vi "auto_light.vi"() -> ()   [LabVIEW 2017]
uses:
  <vilib>/LabVIEW Interface for Arduino/Type Defs/Arduino Resource.ctl
  <vilib>/LabVIEW Interface for Arduino/Type Defs/Board Type.ctl
  <vilib>/LabVIEW Interface for Arduino/LabVIEW Interface for Arduino.lvlib
panel:
  out "机电控制资源1":T1={"VISA resource"="", "Board Type"=enum."Uno", "Connection Type"=enum."USB / Serial", "Bytes Per Packet (15)"=15} caption="机电控制资源"
  out "机电控制报错1":errorcluster caption="机电控制报错"
  in  "?":enum32{"匀光", "标定", "传感器校准", "参数"}(tab)
  in  "红光":bool
  in  "退出程序":bool
  in  "连接":bool
  in  "SENSOR":refnum<visa-resource-name>
  in  "PWM2":u8=70
  in  "PWM3":u8=70
  in  "PWM1":u8=70
  in  "PWM5":u8=70
  in  "PWM4":u8=70
  in  "PWM6":u8=70
  in  "PWM7":u8=70
  in  "PWM8":u8=70
  in  "PWM9":u8=70
  out "光强2":dbl format="%#.2f"
  out "光强1":dbl format="%#.2f"
  out "光强3":dbl format="%#.2f"
  out "光强4":dbl format="%#.2f"
  out "光强5":dbl format="%#.2f"
  out "光强6":dbl format="%#.2f"
  out "光强7":dbl format="%#.2f"
  out "光强8":dbl format="%#.2f"
  out "光强9":dbl format="%#.2g"
  in  "目标光强":dbl
  in  "紫光":bool
  in  "自动匀光":bool
  out "平均光强":dbl caption="目标光强"
  in  "取消匀光":bool
  in  "精度":dbl caption="目标光强"
  in  "LIGHT":refnum<visa-resource-name>
  in  "开始标定":bool
  out "进度条":string
  out "c":string
  out "b":string
  out "a":string
  out "?":string
  out "?":string
  out "?":string
  out "?":string
  out "?":string
  out "?":string
  out "?":string
  out "?":string
  out "?":string
  out "?":string
  out "?":string
  out "?":string
  out "?":string
  out "?":string
  out "?":string
  out "?":string
  out "?":string
  out "?":string
  out "?":string
  out "?":string
  out "?":string
  out "?":string
  out "?":string
  out "?":string
  out "c":string
  out "b":string
  out "a":string
  out "?":string
  out "?":string
  out "?":string
  out "?":string
  out "?":string
  out "?":string
  out "?":string
  out "?":string
  out "?":string
  out "?":string
  out "?":string
  out "?":string
  out "?":string
  out "?":string
  out "?":string
  out "?":string
  out "?":string
  out "?":string
  out "?":string
  out "?":string
  out "?":string
  out "?":string
  out "?":string
  out "?":string
  out "?":string
  out "?":string
  out "?":string
  out "?":string
  out "?":string
  out "?":string
  out "?":string
  out "?":string
  out "?":string
  out "c":string
  out "b":string
  out "a":string
  out "?":string
  out "?":string
  out "?":string
  out "?":string
  out "?":string
  out "?":string
  out "?":string
  out "?":string
  out "?":string
  out "?":string
  out "?":string
  out "?":string
  out "?":string
  out "?":string
  out "?":string
  out "?":string
  out "?":string
  out "?":string
  out "?":string
  out "?":string
  out "?":string
  out "?":string
  out "?":string
  out "?":string
  out "?":string
  out "?":string
  out "?":string
  out "?":string
  out "?":string
  out "?":string
  out "?":string
  out "?":string
  out "?":string
  out "c":string
  out "b":string
  out "a":string
  out "?":string
  out "?":string
  out "?":string
  out "?":string
  out "?":string
  out "?":string
  out "?":string
  out "?":string
  out "?":string
  in  "红光能量（0-255）":u8=255
  in  "红光PWM Pin":u8=11
  out "PWM Pins 4":u8[](array[numeric])=[8, 9, 10] caption="PWM Pins 3"
  out "PWM Pins 5":u8[](array[numeric])=[5, 6, 7] caption="PWM Pins 2"
  out "PWM Pins 6":u8[](array[numeric])=[2, 3, 4] caption="PWM Pins"
  # "S25"
  # "S13"
  # "S1"
  # "S37"
  # "S26"
  # "S14"
  # "S2"
  # "S27"
  # "S15"
  # "S3"
  # "S28"
  # "S16"
  # "S4"
  # "S29"
  # "S17"
  # "S5"
  # "S30"
  # "S18"
  # "S6"
  # "S31"
  # "S19"
  # "S7"
  # "S32"
  # "S20"
  # "S8"
  # "S33"
  # "S21"
  # "S9"
  # "S34"
  # "S22"
  # "S10"
  # "S35"
  # "S23"
  # "S11"
  # "S36"
  # "S24"
  # "S12"
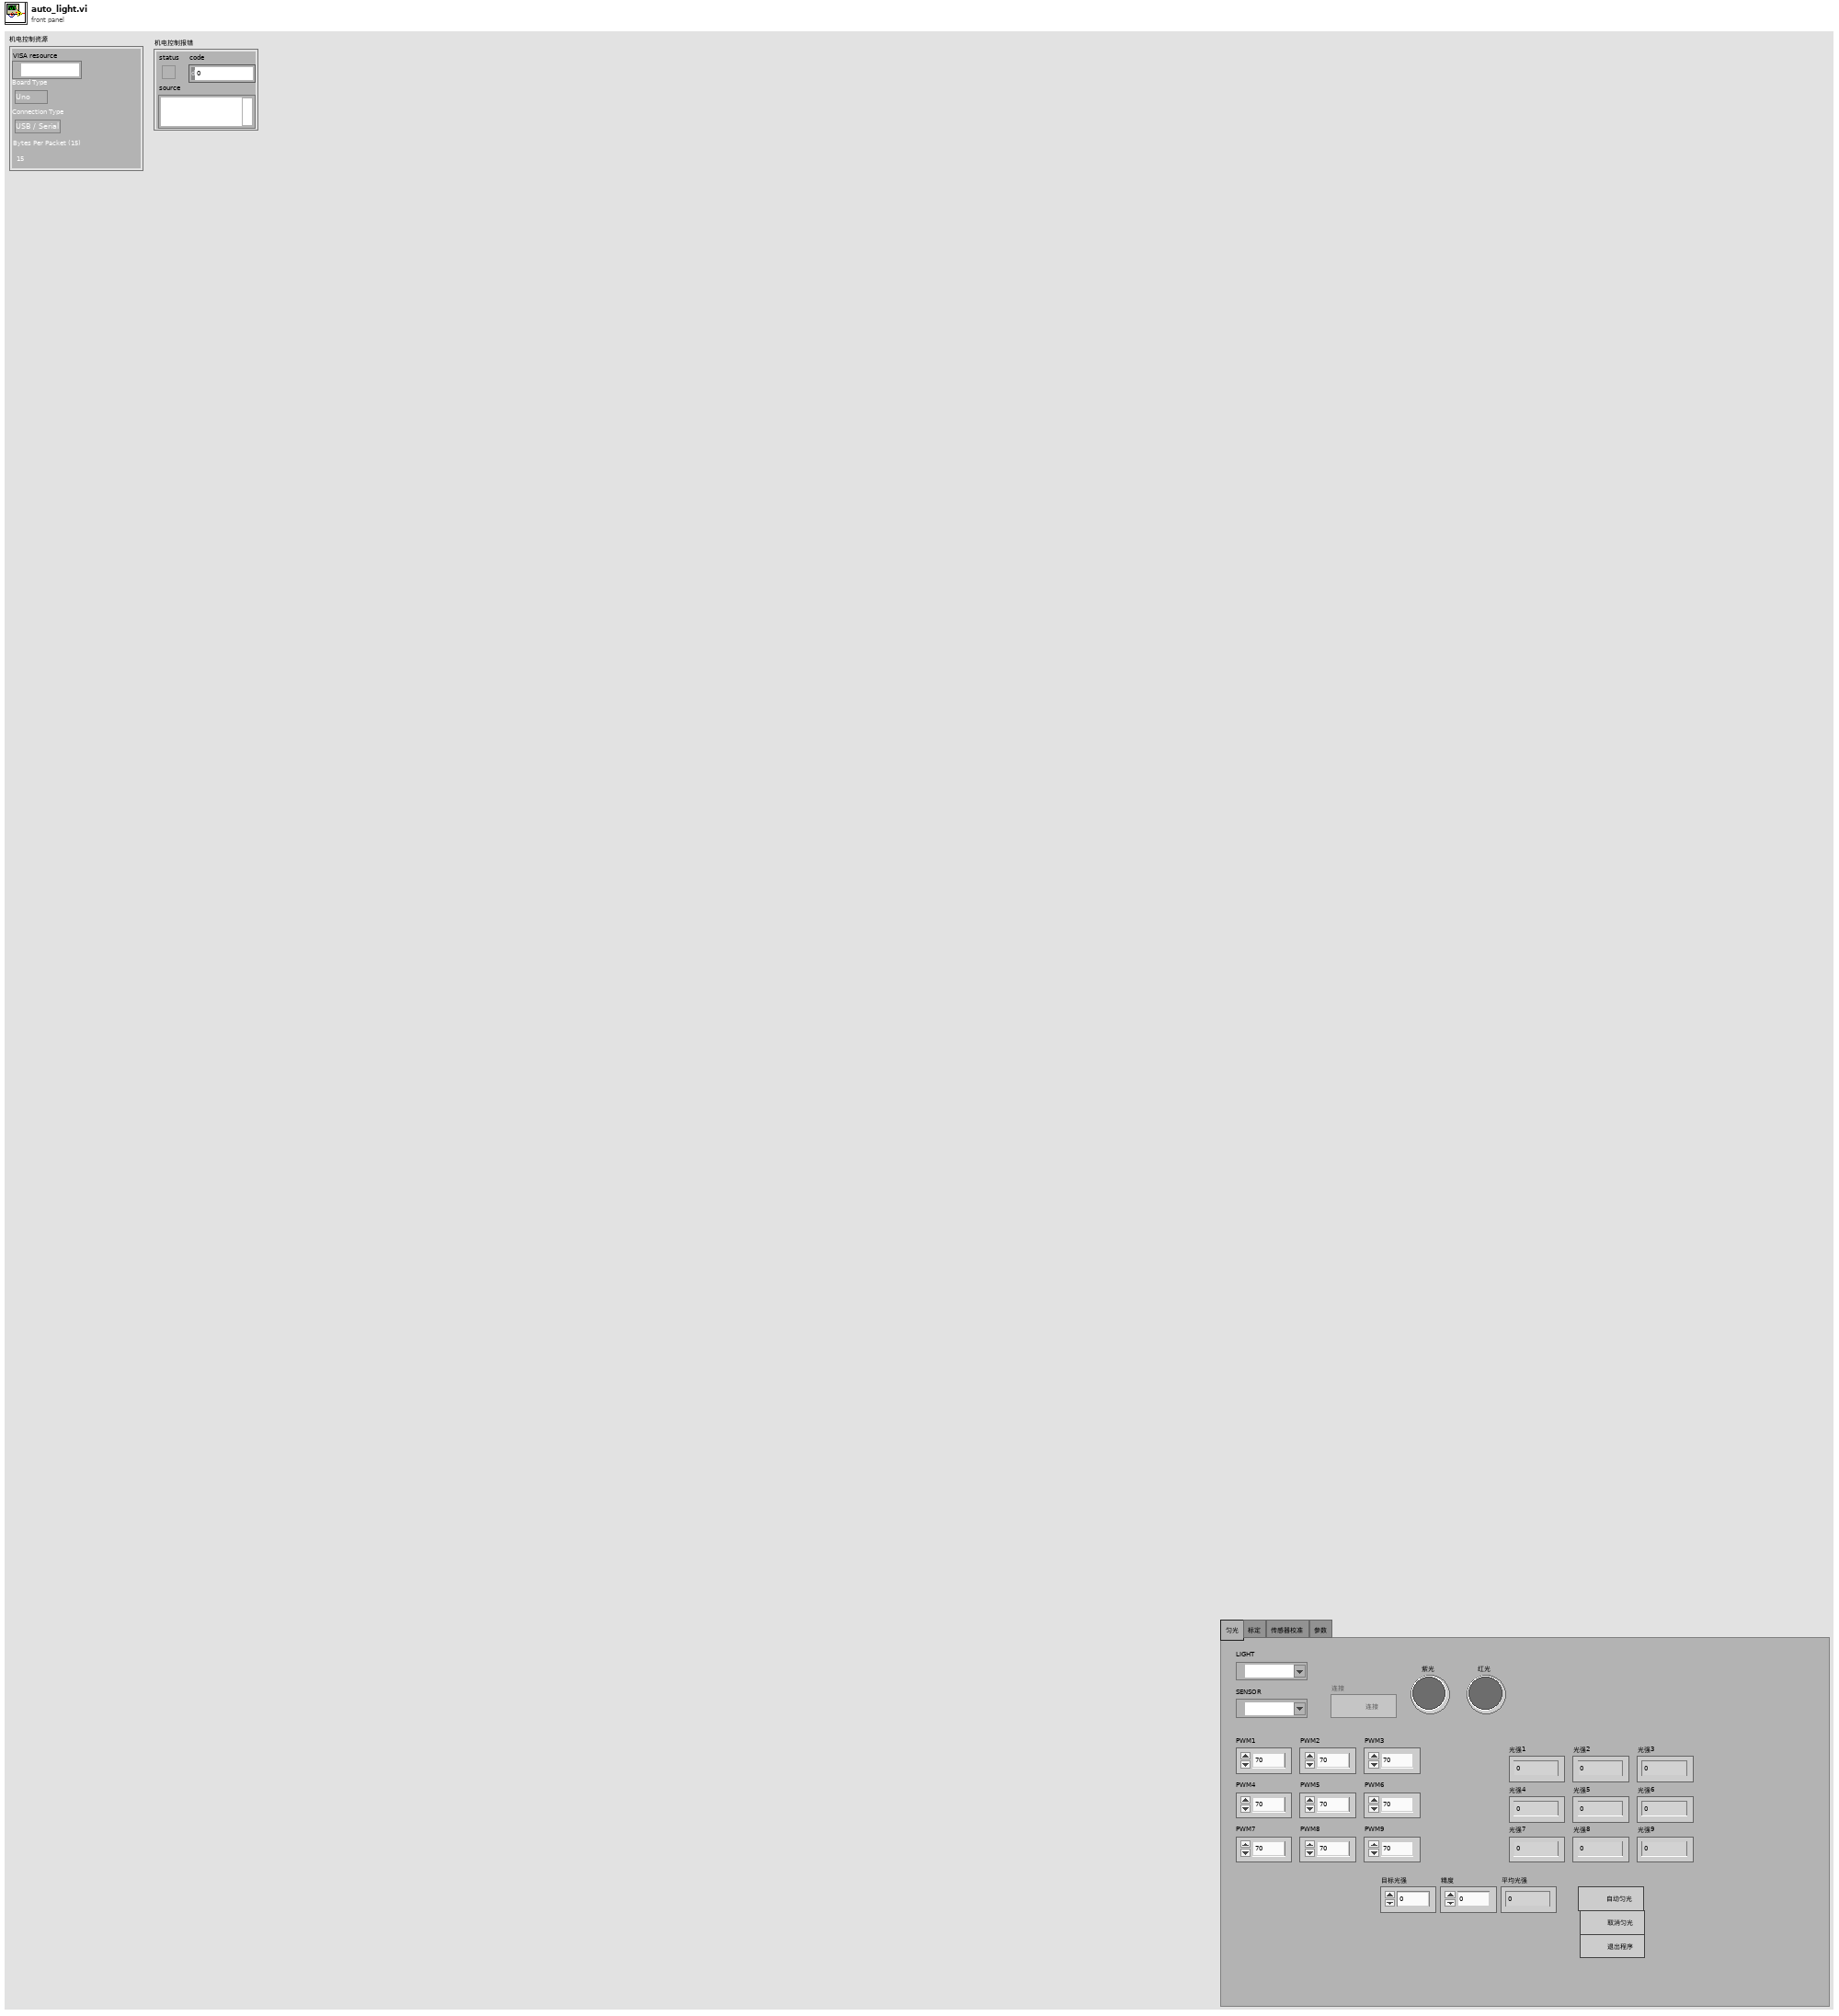
[diagram p1: front panel]
types:
  T1 = typedef "LabVIEW Interface for Arduino.lvlib/Arduino Resource.ctl" = cluster{"VISA resource":refnum<visa-resource-name>, "Board Type":T2, "Connection Type":enum8{"USB / Serial"}, "Bytes Per Packet (15)":u8}
  T2 = typedef "LabVIEW Interface for Arduino.lvlib/Board Type.ctl" = enum16{"Uno", "Dimuelanove w/Atmega 328", "Mega 2560"}
  T3 = enum8{"Enabled", "Disabled", "Disabled and Grayed Out"}
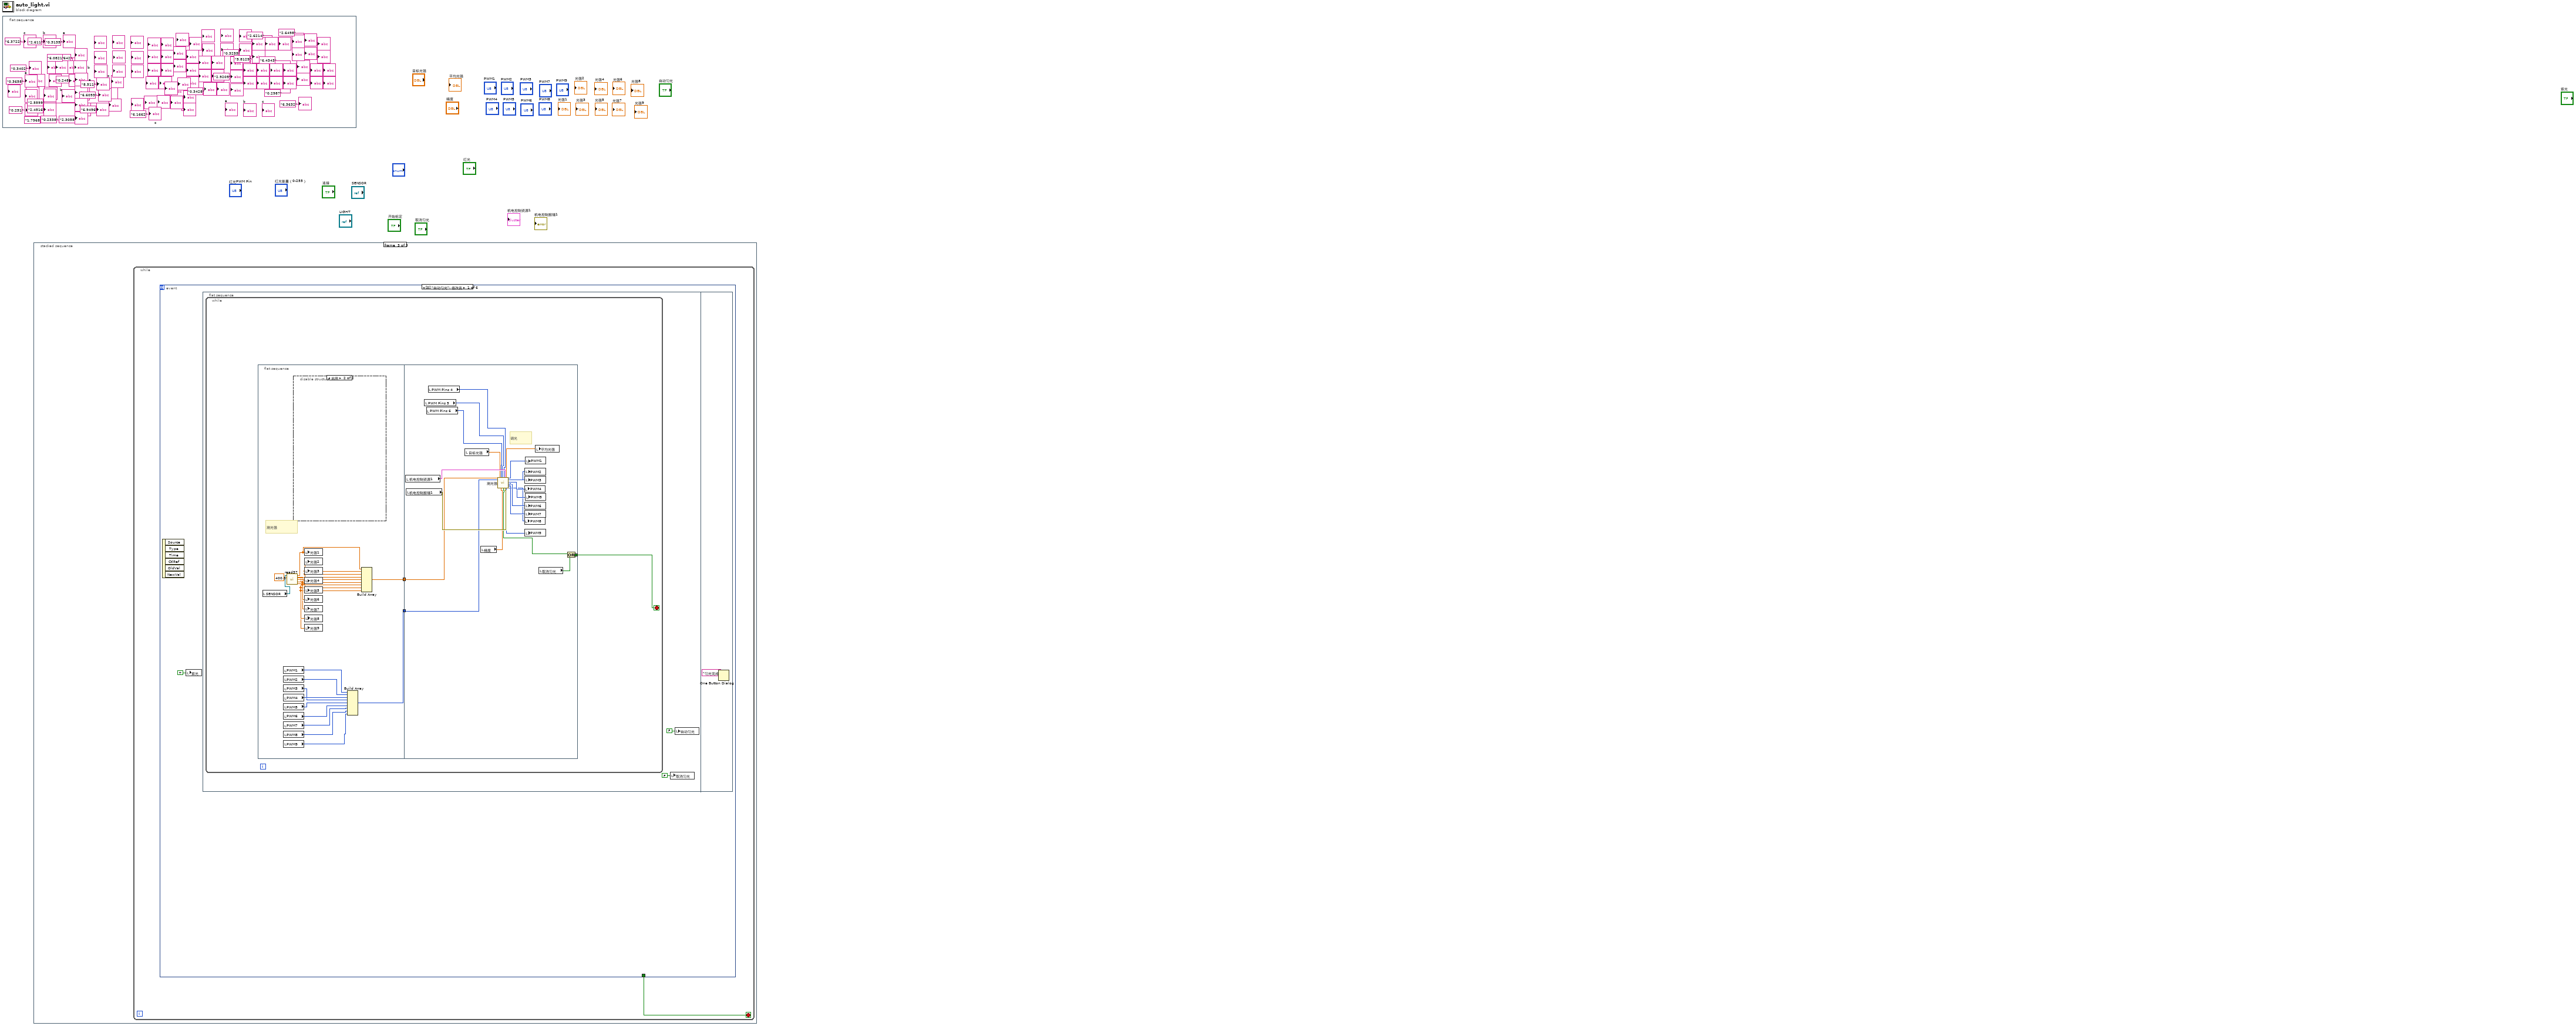
[diagram p0: block diagram]
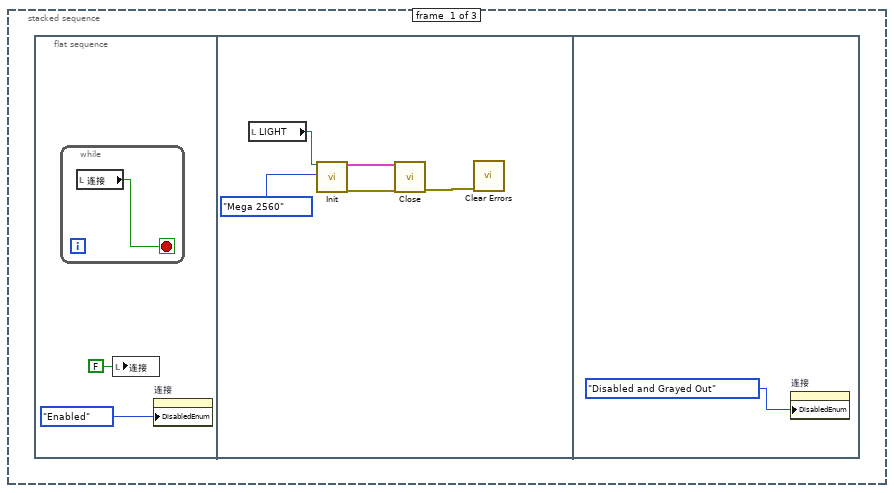
[diagram p2: hidden frame]
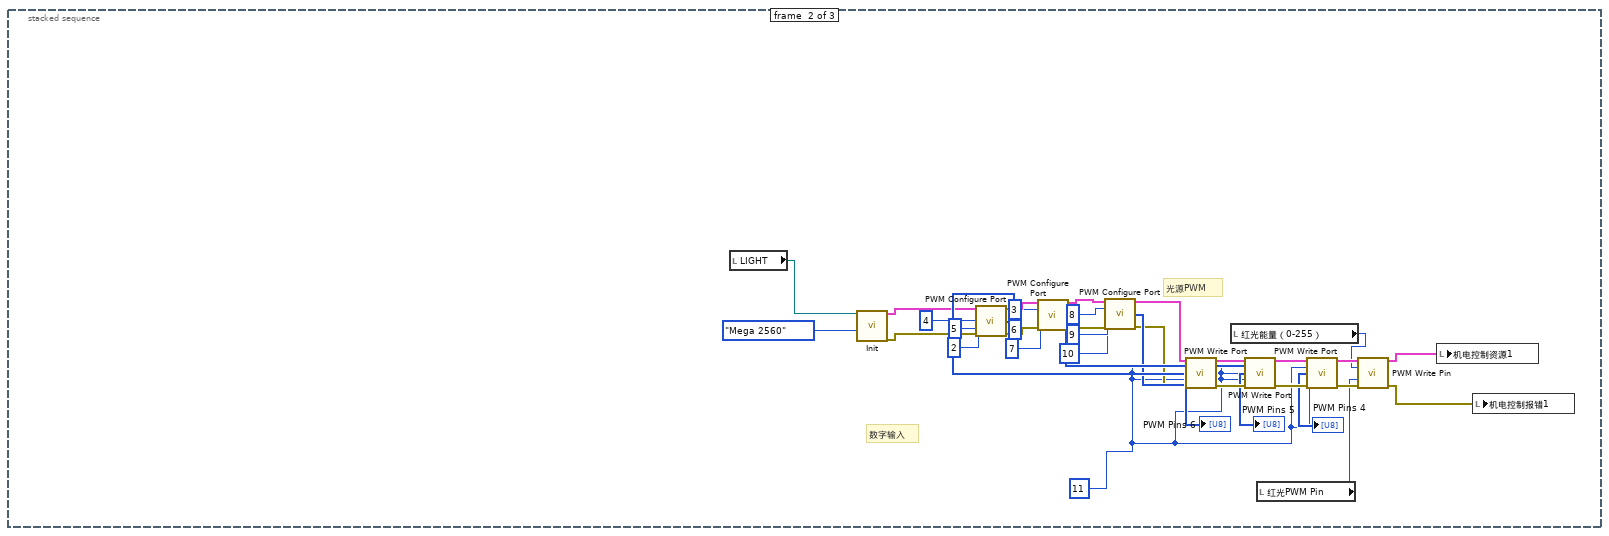
[diagram p3: hidden frame]
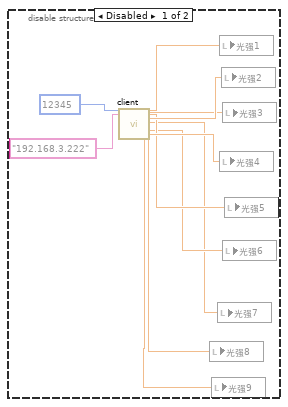
[diagram p4: hidden frame]
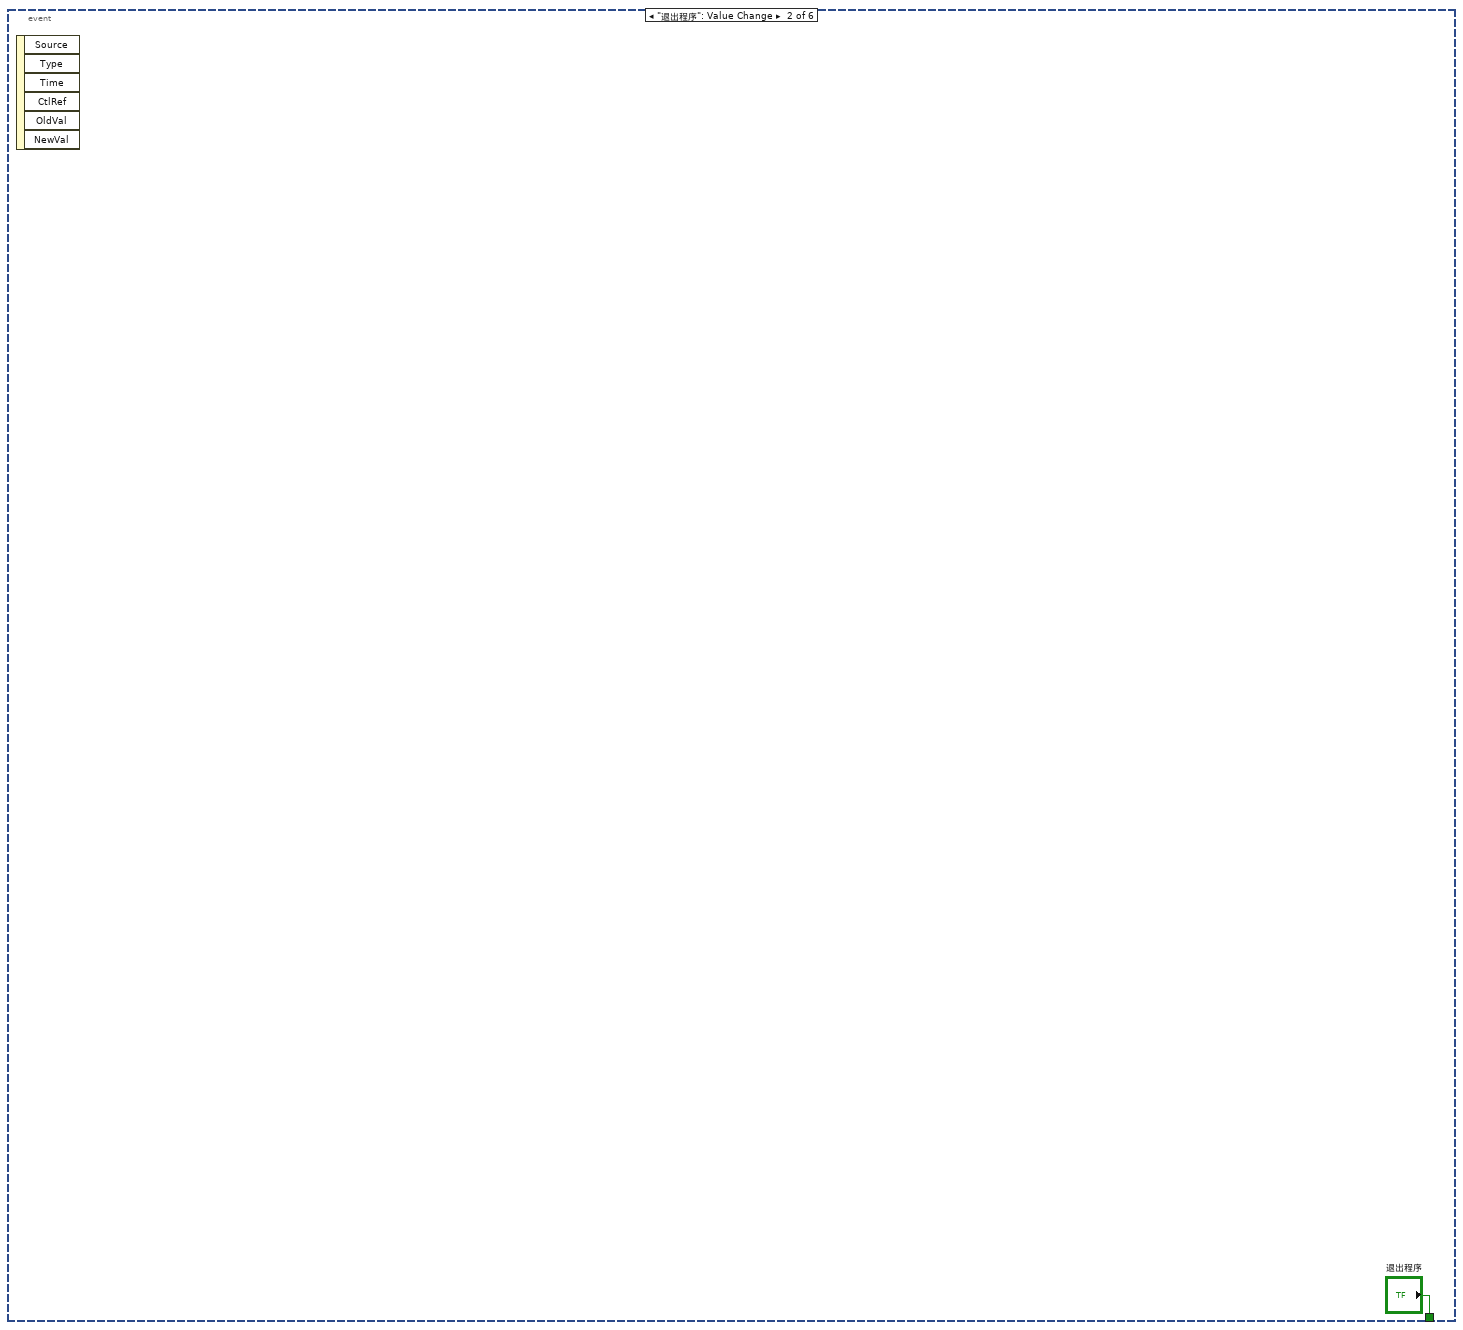
[diagram p5: hidden frame]
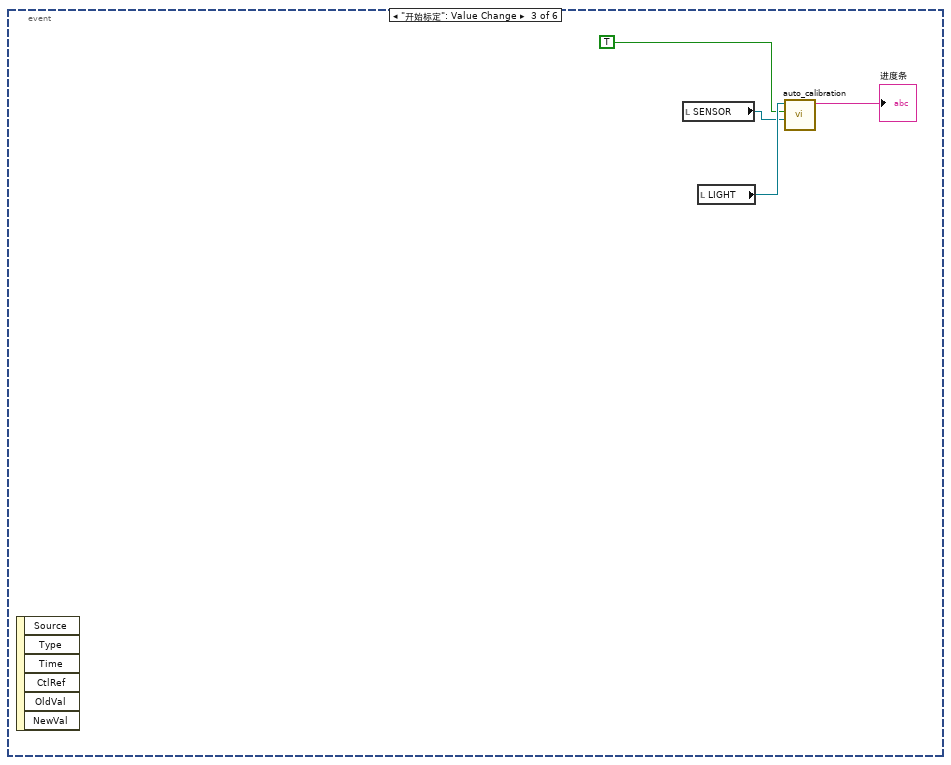
[diagram p6: hidden frame]
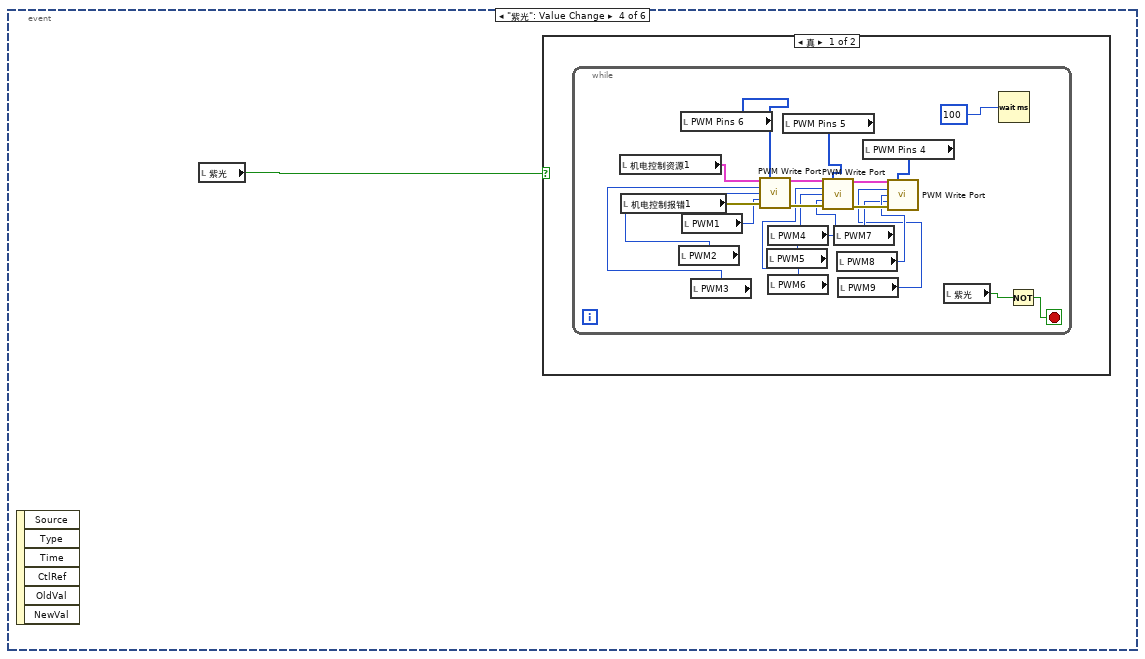
[diagram p7: hidden frame]
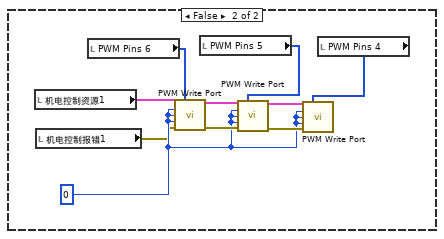
[diagram p8: hidden frame]
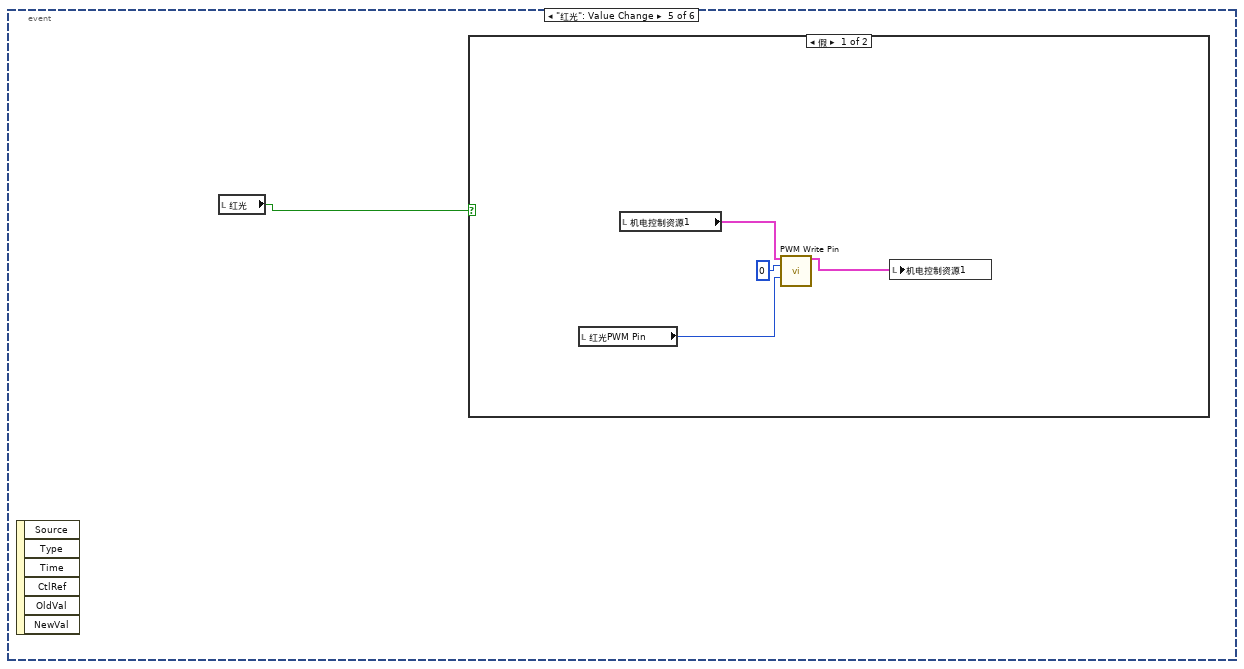
[diagram p9: hidden frame]
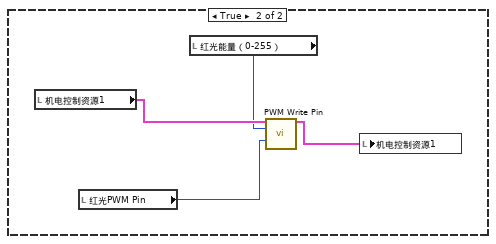
[diagram p10: hidden frame]
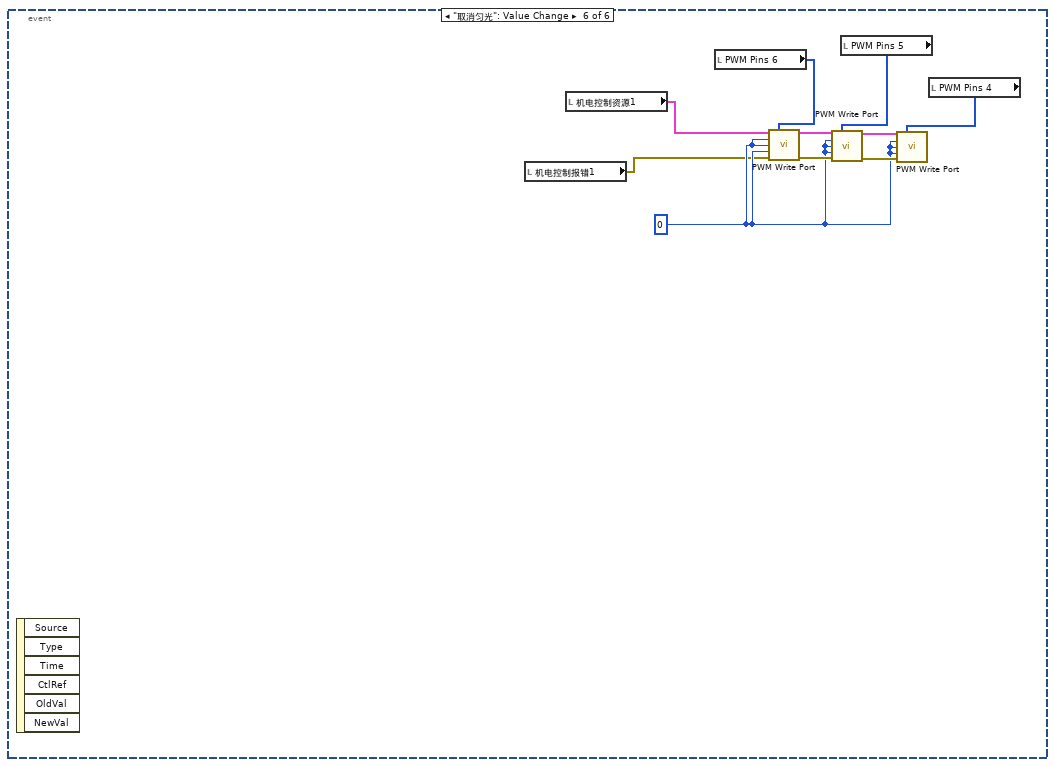
[diagram p11: hidden frame]
diagram:
  n1 = flat-sequence {
    frame #0 {
      "a" <- "0.3135" ("a")
      "c" <- "6.3722" ("c")
      "b" <- "2.611" ("b")
      "a" <- "0.3658" ("a")
      "b" <- "1.7968" ("b")
      "c" <- "8.511" ("c")
      "?" <- "0.251"
      "?" <- "2.4516"
      "?" <- "6.6093"
      "a" <- "0.248" ("a")
      "b" <- "2.7642" ("b")
      "?" <- "2.5599"
      "?" <- "0.3402"
      "?" <- "6.0821"
      "?" <- "0.2338"
      "?" <- "2.3058"
      "?" <- "6.9496"
      "c" <- "6.1662" ("c")
      "?" <- "5.8129"
      "?" <- "2.9209"
      "?" <- "0.3428"
      "?" <- "6.3632"
      "?" <- "2.6214"
      "?" <- "0.3255"
      "?" <- "6.4343"
      "?" <- "2.6498"
      "?" <- "0.2987"
    }
  }
  n2 = stacked-sequence {
    frame #0 {
      n3 = flat-sequence {
        frame #0 {
          n4 = while {
            stop <- w30 stop-if-true
            n5 = local read "连接"() -> (w30:bool)
          }
          n6 = local write "连接"(FALSE ("连接")) -> ()
          n7 = property on="连接" class="Bool (严格)"("DisabledEnum"=T3."Enabled" ("禁用")) -> ()  [unwired: 2 in, 2 out]
        }
        frame #1 {
          n8 = local read "LIGHT"() -> (w31:refnum<visa-resource-name>)
          n9 = call <vilib>:"Init.vi"("VISA resource"=w31, "Board Type (Uno)"=Board_Type."Mega 2560") -> ("Arduino Resource"=w35:T1, "error out"=w34:errorcluster)  [unwired: 16 in]
          n10 = call <vilib>:"Close.vi"("Arduino Resource"=w35, "error in"=w34) -> ("error out"=w33:errorcluster)  [unwired: 13 in]
          n11 = call <vilib>:"Clear Errors.vi"("error in (no error)"=w33) -> ()  [unwired: 5 in, 2 out]
        }
        frame #2 {
          n12 = property on="连接" class="Bool (严格)"("DisabledEnum"=T3."Disabled and Grayed Out" ("禁用")) -> ()  [unwired: 2 in, 2 out]
        }
      }
    }
    frame #1 {
      w40 = 11
      # "数字输入"
      # "光源PWM"
      n13 = local read "LIGHT"() -> (w39:refnum<visa-resource-name>)
      n14 = call <vilib>:"Init.vi"("VISA resource"=w39, "Board Type (Uno)"=Board_Type."Mega 2560") -> ("Arduino Resource"=w42:T1, "error out"=w41:errorcluster)  [unwired: 16 in]
      n15 = call <vilib>:"PWM Configure Port.vi"("Arduino Resource"=w42, "PWM Pin (3)"=u8 4, "PWM Pin (5)"=u8 5, "PWM Pin (6)"=u8 2, "error in"=w41) -> ("Arduino Resource"=w68:T1, "PWM Pins"=w51:u8[], "error out"=w67:errorcluster)  [unwired: 8 in]
      n16 = call <vilib>:"PWM Configure Port.vi"("Arduino Resource"=w68, "PWM Pin (3)"=u8 3, "PWM Pin (5)"=u8 6, "PWM Pin (6)"=u8 7, "error in"=w67) -> ("Arduino Resource"=w53:T1, "PWM Pins"=w50:u8[], "error out"=w52:errorcluster)  [unwired: 8 in]
      n17 = call <vilib>:"PWM Configure Port.vi"("Arduino Resource"=w53, "PWM Pin (3)"=u8 8, "PWM Pin (5)"=u8 9, "PWM Pin (6)"=u8 10, "error in"=w52) -> ("Arduino Resource"=w48:T1, "PWM Pins"=w49:u8[], "error out"=w47:errorcluster)  [unwired: 8 in]
      n18 = call <vilib>:"PWM Write Port.vi"("Arduino Resource"=w48, "PWM Pins"=w51, "PWM 0 (0-255)"=w40, "PWM 1 (0-255)"=w40, "PWM 2 (0-255)"=w40, "error in"=w47) -> ("Arduino Resource"=w60:T1, "PWM Pins"=→"PWM Pins 6":u8[], "error out"=w59:errorcluster)  [unwired: 7 in]
      n19 = local read "红光能量（0-255）"() -> (w43:u8)
      n20 = call <vilib>:"PWM Write Port.vi"("Arduino Resource"=w60, "PWM Pins"=w50, "PWM 0 (0-255)"=w40, "PWM 1 (0-255)"=w40, "PWM 2 (0-255)"=w40, "error in"=w59) -> ("Arduino Resource"=w58:T1, "PWM Pins"=→"PWM Pins 5":u8[], "error out"=w57:errorcluster)  [unwired: 7 in]
      n21 = local read "红光PWM Pin"() -> (w44:u8)
      n22 = call <vilib>:"PWM Write Port.vi"("Arduino Resource"=w58, "PWM Pins"=w49, "PWM 0 (0-255)"=w40, "PWM 1 (0-255)"=w40, "PWM 2 (0-255)"=w40, "error in"=w57) -> ("Arduino Resource"=w46:T1, "PWM Pins"=→"PWM Pins 4":u8[], "error out"=w45:errorcluster)  [unwired: 7 in]
      n23 = call <vilib>:"PWM Write Pin.vi"("Arduino Resource"=w46, "Duty Cycle (0 - 255)"=w43, "PWM Pin (3)"=w44, "error in"=w45) -> ("Arduino Resource"=w38:T1, "error out"=w37:errorcluster)  [unwired: 10 in]
      n24 = local write "机电控制资源1"(w38) -> ()
      n25 = local write "机电控制报错1"(w37) -> ()
    }
    frame #2 {
      n26 = while {
        stop <- w73 stop-if-true
        n27 = event shown="[0] \"自动匀光\": 值改变" {
          selector: _ -> [_ _ _ _ _ _]
          dyn-events: _ -> [_ _ _ _ _ _]
          timeout: _ -> [_ _ _ _ _ _]
          tunnel: [_ "退出程序" _ _ _ _] -> w73
          event "自动匀光": Value Change {
            n28 = event-data() -> ()  [unwired: 1 in, 6 out]
            n29 = local write "紫光"(TRUE ("紫光")) -> ()
            n30 = flat-sequence {
              frame #0 {
                n31 = while {
                  stop <- w79 stop-if-true
                  n32 = flat-sequence {
                    tunnel: [w101] -> w78
                    tunnel: [w100] -> w77
                    tunnel: [w118] -> w79
                    tunnel: w78 -> [w114]
                    tunnel: w77 -> [w113]
                    frame #0 {
                      # "测光强"
                      n33 = local read "SENSOR"() -> (w99:refnum<visa-resource-name>)
                      n34 = local read "PWM1"() -> (w88:u8)
                      n35 = local read "PWM2"() -> (w87:u8)
                      n36 = local read "PWM3"() -> (w86:u8)
                      n37 = local read "PWM4"() -> (w85:u8)
                      n38 = local read "PWM5"() -> (w84:u8)
                      n39 = local read "PWM6"() -> (w83:u8)
                      n40 = local read "PWM7"() -> (w82:u8)
                      n41 = local read "PWM8"() -> (w81:u8)
                      n42 = local read "PWM9"() -> (w80:u8)
                      n43 = call "read37.vi"("VISA资源名称"=w99, "Interval_ms"=400.0) -> ("SENSOR8"=w90:dbl, "SENSOR6"=w92:dbl, "SENSOR1"=w97:dbl, "SENSOR2"=w96:dbl, "SENSOR3"=w95:dbl, "SENSOR4"=w94:dbl, "SENSOR9"=w89:dbl, "SENSOR7"=w91:dbl, "SENSOR5"=w93:dbl)  [unwired: 5 in]
                      n44 = disable-structure shown="启用" {
                        frame Disabled {
                          n45 = call "client.vi"("远程端口或服务名称"=u16 12345, "地址"="192.168.3.222") -> ("num9"=w102:dbl, "num1"=w111:dbl, "num2"=w107:dbl, "num3"=w110:dbl, "num4"=w105:dbl, "num5"=w109:dbl, "num7"=w106:dbl, "num6"=w108:dbl, "num8"=w103:dbl)  [unwired: 17 in]
                          n46 = local write "光强8"(w103) -> ()
                          n47 = local write "光强9"(w102) -> ()
                          n48 = local write "光强7"(w105) -> ()
                          n49 = local write "光强1"(w111) -> ()
                          n50 = local write "光强4"(w108) -> ()
                          n51 = local write "光强2"(w110) -> ()
                          n52 = local write "光强3"(w109) -> ()
                          n53 = local write "光强6"(w106) -> ()
                          n54 = local write "光强5"(w107) -> ()
                        }
                        frame Enabled {
                        }
                      }
                      n55 = local write "光强1"(w97) -> ()
                      n56 = local write "光强2"(w96) -> ()
                      n57 = local write "光强3"(w95) -> ()
                      n58 = local write "光强4"(w94) -> ()
                      n59 = local write "光强5"(w93) -> ()
                      n60 = local write "光强6"(w92) -> ()
                      n61 = local write "光强7"(w91) -> ()
                      n62 = local write "光强8"(w90) -> ()
                      n63 = local write "光强9"(w89) -> ()
                      n64 = Build Array(w88, w87, w86, w85, w84, w83, w82, w81, w80) -> (w100:u8[])
                      n65 = Build Array(w97, w96, w95, w94, w93, w92, w91, w90, w89) -> (w101:dbl[])
                    }
                    frame #1 {
                      # "调光"
                      n66 = local read "机电控制资源1"() -> (w133:T1)
                      n67 = local read "机电控制报错1"() -> (w134:errorcluster)
                      n68 = local read "PWM Pins 5"() -> (w116:u8[])
                      n69 = local read "PWM Pins 6"() -> (w117:u8[])
                      n70 = local read "PWM Pins 4"() -> (w115:u8[])
                      n71 = local read "目标光强"() -> (w119:dbl)
                      n72 = local read "精度"() -> (w130:dbl)
                      n73 = call "测光强.vi"("光强数组"=w114, "pwm（更新前）"=w113, "目标光强"=w119, "PWM Pins"=w117, "精度"=w130, "PWM Pins 2"=w116, "PWM Pins 3"=w115, "光源控制资源"=w133, "光源控制报错"=w134) -> ("停止"=w132:bool, "平均光强"=w120:dbl, "PWM9"=w124:u8, "PWM1"=w121:u8, "PWM2"=w122:u8, "PWM3"=w123:u8, "PWM4"=w129:u8, "PWM5"=w128:u8, "PWM6"=w127:u8, "PWM7"=w126:u8, "PWM8"=w125:u8)  [unwired: 8 in]
                      n74 = local write "PWM4"(w129) -> ()
                      n75 = local write "PWM8"(w125) -> ()
                      n76 = local write "PWM2"(w122) -> ()
                      n77 = local write "PWM3"(w123) -> ()
                      n78 = local write "PWM6"(w127) -> ()
                      n79 = local write "PWM7"(w126) -> ()
                      n80 = local write "PWM9"(w124) -> ()
                      n81 = local write "PWM1"(w121) -> ()
                      n82 = local write "PWM5"(w128) -> ()
                      n83 = local write "平均光强"(w120) -> ()
                      n84 = local read "取消匀光"() -> (w131:bool)
                      n85 = Or(x=w132, y=w131) -> (x .or. y?=w118:bool)
                    }
                  }
                }
                n86 = local write "取消匀光"(FALSE ("取消匀光")) -> ()
                n87 = local write "自动匀光"(FALSE ("自动匀光")) -> ()
              }
              frame #1 {
                n88 = One Button Dialog(message="匀光完成" ("消息")) -> ()  [unwired: 1 in, 1 out]
              }
            }
          }
          event "退出程序": Value Change {
            n89 = event-data() -> ()  [unwired: 1 in, 6 out]
          }
          event "开始标定": Value Change {
            n90 = event-data() -> ()  [unwired: 1 in, 6 out]
            n91 = local read "SENSOR"() -> (w139:refnum<visa-resource-name>)
            n92 = local read "LIGHT"() -> (w140:refnum<visa-resource-name>)
            n93 = call "auto_calibration.vi"("VISA传感器面板"=w139, "启动"=TRUE, "VISA灯板"=w140) -> ("进度条"=→"进度条":string)  [unwired: 8 in]
          }
          event "紫光": Value Change {
            n94 = event-data() -> ()  [unwired: 1 in, 6 out]
            n95 = local read "紫光"() -> (w141:bool)
            n96 = case shown="真" w141 {
              frame True {
                n97 = while {
                  stop <- w154 stop-if-true
                  n98 = local read "机电控制资源1"() -> (w152:T1)
                  n99 = local read "机电控制报错1"() -> (w151:errorcluster)
                  n100 = local read "PWM2"() -> (w156:u8)
                  n101 = local read "PWM Pins 6"() -> (w144:u8[])
                  n102 = local read "PWM1"() -> (w150:u8)
                  n103 = local read "PWM3"() -> (w149:u8)
                  n104 = call <vilib>:"PWM Write Port.vi"("Arduino Resource"=w152, "PWM Pins"=w144, "PWM 0 (0-255)"=w149, "PWM 1 (0-255)"=w156, "PWM 2 (0-255)"=w150, "error in"=w151) -> ("Arduino Resource"=w162:T1, "error out"=w161:errorcluster)  [unwired: 7 in, 1 out]
                  n105 = local read "PWM5"() -> (w157:u8)
                  n106 = local read "PWM4"() -> (w148:u8)
                  n107 = local read "PWM6"() -> (w147:u8)
                  n108 = local read "PWM Pins 5"() -> (w143:u8[])
                  n109 = call <vilib>:"PWM Write Port.vi"("Arduino Resource"=w162, "PWM Pins"=w143, "PWM 0 (0-255)"=w147, "PWM 1 (0-255)"=w157, "PWM 2 (0-255)"=w148, "error in"=w161) -> ("Arduino Resource"=w160:T1, "error out"=w159:errorcluster)  [unwired: 7 in, 1 out]
                  n110 = local read "PWM7"() -> (w146:u8)
                  n111 = local read "PWM8"() -> (w158:u8)
                  n112 = local read "PWM9"() -> (w145:u8)
                  n113 = local read "PWM Pins 4"() -> (w142:u8[])
                  n114 = call <vilib>:"PWM Write Port.vi"("Arduino Resource"=w160, "PWM Pins"=w142, "PWM 0 (0-255)"=w145, "PWM 1 (0-255)"=w158, "PWM 2 (0-255)"=w146, "error in"=w159) -> ()  [unwired: 7 in, 3 out]
                  n115 = local read "紫光"() -> (w155:bool)
                  n116 = Wait (ms)(milliseconds to wait=u32 100 ("等待时间（毫秒）")) -> ()  [unwired: 1 out]
                  n117 = Not(x=w155) -> (.not. x?=w154:bool)
                }
              }
              frame False {
                w168 = u8 0
                n118 = local read "机电控制资源1"() -> (w167:T1)
                n119 = local read "机电控制报错1"() -> (w166:errorcluster)
                n120 = local read "PWM Pins 6"() -> (w165:u8[])
                n121 = call <vilib>:"PWM Write Port.vi"("Arduino Resource"=w167, "PWM Pins"=w165, "PWM 0 (0-255)"=w168, "PWM 1 (0-255)"=w168, "PWM 2 (0-255)"=w168, "error in"=w166) -> ("Arduino Resource"=w172:T1, "error out"=w171:errorcluster)  [unwired: 7 in, 1 out]
                n122 = local read "PWM Pins 5"() -> (w164:u8[])
                n123 = call <vilib>:"PWM Write Port.vi"("Arduino Resource"=w172, "PWM Pins"=w164, "PWM 0 (0-255)"=w168, "PWM 1 (0-255)"=w168, "PWM 2 (0-255)"=w168, "error in"=w171) -> ("Arduino Resource"=w170:T1, "error out"=w169:errorcluster)  [unwired: 7 in, 1 out]
                n124 = local read "PWM Pins 4"() -> (w163:u8[])
                n125 = call <vilib>:"PWM Write Port.vi"("Arduino Resource"=w170, "PWM Pins"=w163, "PWM 0 (0-255)"=w168, "PWM 1 (0-255)"=w168, "PWM 2 (0-255)"=w168, "error in"=w169) -> ()  [unwired: 7 in, 3 out]
              }
            }
          }
          event "红光": Value Change {
            n126 = event-data() -> ()  [unwired: 1 in, 6 out]
            n127 = local read "红光"() -> (w173:bool)
            n128 = case shown="假" w173 {
              frame False {
                n129 = local read "红光PWM Pin"() -> (w174:u8)
                n130 = local read "机电控制资源1"() -> (w176:T1)
                n131 = call <vilib>:"PWM Write Pin.vi"("Arduino Resource"=w176, "Duty Cycle (0 - 255)"=u8 0, "PWM Pin (3)"=w174) -> ("Arduino Resource"=w175:T1)  [unwired: 11 in, 1 out]
                n132 = local write "机电控制资源1"(w175) -> ()
              }
              frame True {
                n133 = local read "机电控制资源1"() -> (w181:T1)
                n134 = local read "红光PWM Pin"() -> (w178:u8)
                n135 = local read "红光能量（0-255）"() -> (w179:u8)
                n136 = call <vilib>:"PWM Write Pin.vi"("Arduino Resource"=w181, "Duty Cycle (0 - 255)"=w179, "PWM Pin (3)"=w178) -> ("Arduino Resource"=w180:T1)  [unwired: 11 in, 1 out]
                n137 = local write "机电控制资源1"(w180) -> ()
              }
            }
          }
          event "取消匀光": Value Change {
            w187 = u8 0
            n138 = event-data() -> ()  [unwired: 1 in, 6 out]
            n139 = local read "机电控制报错1"() -> (w185:errorcluster)
            n140 = local read "机电控制资源1"() -> (w186:T1)
            n141 = local read "PWM Pins 6"() -> (w184:u8[])
            n142 = call <vilib>:"PWM Write Port.vi"("Arduino Resource"=w186, "PWM Pins"=w184, "PWM 0 (0-255)"=w187, "PWM 1 (0-255)"=w187, "PWM 2 (0-255)"=w187, "error in"=w185) -> ("Arduino Resource"=w188:T1, "error out"=w189:errorcluster)  [unwired: 7 in, 1 out]
            n143 = local read "PWM Pins 5"() -> (w183:u8[])
            n144 = call <vilib>:"PWM Write Port.vi"("Arduino Resource"=w188, "PWM Pins"=w183, "PWM 0 (0-255)"=w187, "PWM 1 (0-255)"=w187, "PWM 2 (0-255)"=w187, "error in"=w189) -> ("Arduino Resource"=w190:T1, "error out"=w191:errorcluster)  [unwired: 7 in, 1 out]
            n145 = local read "PWM Pins 4"() -> (w182:u8[])
            n146 = call <vilib>:"PWM Write Port.vi"("Arduino Resource"=w190, "PWM Pins"=w182, "PWM 0 (0-255)"=w187, "PWM 1 (0-255)"=w187, "PWM 2 (0-255)"=w187, "error in"=w191) -> ()  [unwired: 7 in, 3 out]
          }
        }
      }
    }
  }
